vi "int.vi"() -> ()   [LabVIEW 2016]
uses:
  <vilib>/imath/engines/lvmath2/RunTimeEngine/NodeEndStatement/NIMS_NodeEndStatement_Output.vi
  <instcachedir>/0/NIMS_NodeEndStatement_Output_53EC0D466D134D7ABD903AC30B43404B.lvgen/NIMS_NodeEndStatement_Output_53EC0D466D134D7ABD903AC30B43404B_011.vi
  <vilib>/imath/engines/lvmath2/RunTimeEngine/ErrorHandling/NIMS_Finalize Error.vi
  <vilib>/imath/engines/lvmath2/RunTimeEngine/VariableToken/NIMS_VariableToken_CondDefined.vi
  <instcachedir>/0/NIMS_VariableToken_CondDefined_06E9DA95BD4D46A6BA55EC651A891960.lvgen/NIMS_VariableToken_CondDefined_06E9DA95BD4D46A6BA55EC651A891960_008.vi
  <vilib>/imathl/engines/lvmath/Functions/Error Handling/Create Error.vi
  <vilib>/imath/engines/lvmath/Functions/Error Handling/MergeErrorsWrapper.vi
  <instcachedir>/0/NIMS_NodeEndStatement_Output_53EC0D466D134D7ABD903AC30B43404B.lvgen/NIMS_NodeEndStatement_Output_53EC0D466D134D7ABD903AC30B43404B_009.vi
panel:
  in  "停止":bool
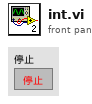
[diagram p1: front panel]
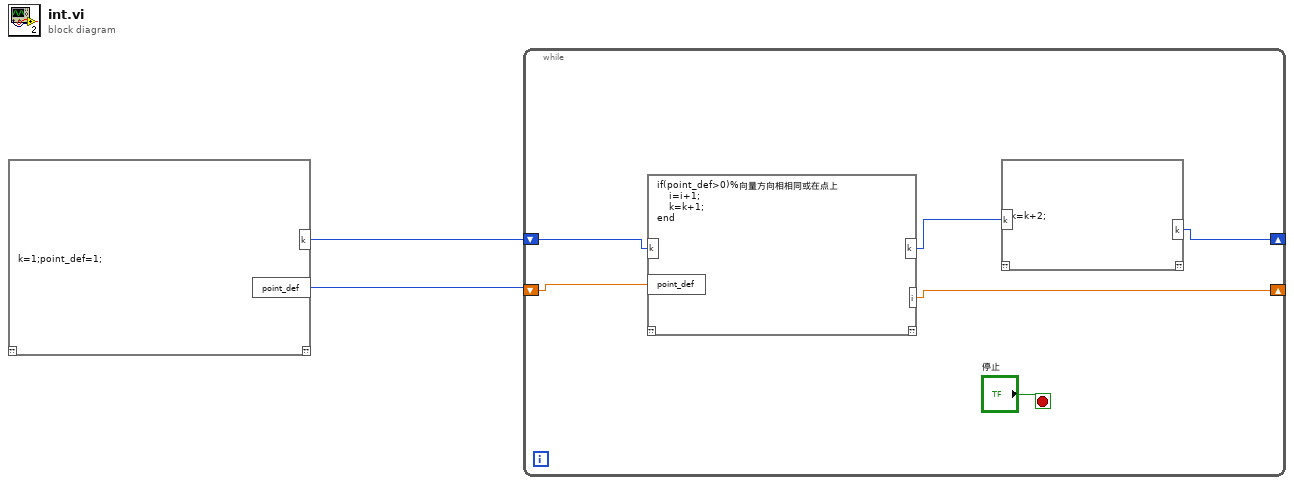
[diagram p0: block diagram]
diagram:
  n1 = mathscript code="k=1;point_def=1;"() -> ("k"=w2:i32, "point_def"=w1:i32)  [unwired: 1 in, 1 out]
  n2 = while {
    shift-right: [w3] -> _
    shift-left: w2 -> [w5]
    shift-right: [w6] -> _
    shift-left: w1 -> [w7]
    stop <- "停止" stop-if-true
    n3 = mathscript code="if(point_def>0)%向量方向相相同或在点上\n    i=i+1;\n    k=k+1;\nend"("k"=w5, "point_def"=w7) -> ("k"=w4:i32, "i"=w6:cdb)  [unwired: 1 in, 1 out]
    n4 = mathscript code="k=k+2;"("k"=w4) -> ("k"=w3:i32)  [unwired: 1 in, 1 out]
  }
